vi "Dashboard Main.vi"() -> ()   [LabVIEW 2018]
uses:
  <vilib>/Utility/miscctls.llb/LVRowAndColumnTypeDef.ctl
  <vilib>/event_ctls.llb/eventvkey.ctl
  <vilib>/Rock Robotics/WPI/Dashboard/WPI_DashboardLogging Global.vi
panel:
  in  "Camera Settings Right":T1={"Frame Rate"=30, "Compression"=30, "Size"=1, "DB Camera Config"=FALSE} {"Frame Rate" scale=1.0..30.0; "Compression" scale=100.0..-1.0; "Size" items=["640x480", "320x240", "160x120"]}
  in  "Camera Name Right":string(combo)="No Camera Selection"
  out "Camera Perf":string
  in  "Camera Settings":T1={"Frame Rate"=30, "Compression"=30, "Size"=1, "DB Camera Config"=FALSE} {"Frame Rate" scale=1.0..30.0; "Compression" scale=100.0..-1.0; "Size" items=["640x480", "320x240", "160x120"]}
  in  "TCP":refnum<k5>
  in  "Rec Mode":enum32{"Stop", "Record", "Playback"}(radio)
  out "Robot IP":string
  out "Image Message":string="Timeout in Camera Communications"
  in  "Dashboard Tab":T2(tab)
  in  "Select Auto":string(combo)="Select Autonomous ..."
  out "NT Connection":bool
  out "Mode":T3(ring)=enum."Auto Disabled"
  out "Right Camera Perf":cluster{"Bandwidth (Mbps)":dbl, "FPS":dbl}
  out "Camera Image Right":T4(plugin-control)
  in  "DB/String 9":string
  in  "DB/String 8":string
  in  "DB/String 7":string
  in  "DB/String 6":string
  in  "DB/String 5":string
  in  "DB/String 4":string
  in  "DB/String 3":string
  in  "DB/String 2":string
  in  "DB/String 1":string
  in  "DB/String 0":string
  in  "DB/Slider 0":dbl(slide) scale=0.0..5.0
  in  "DB/Slider 1":dbl(slide) scale=0.0..5.0
  in  "DB/Slider 2":dbl(slide) scale=0.0..5.0
  in  "DB/Slider 3":dbl(slide) scale=0.0..5.0
  out "DB/LED 3":bool
  out "DB/LED 2":bool
  out "DB/LED 1":bool
  out "DB/LED 0":bool
  in  "DB/Button 3":bool
  in  "DB/Button 2":bool
  in  "DB/Button 1":bool
  in  "DB/Button 0":bool caption="New Name"
  in  "Test Slider":dbl(slide) scale=0.0..100.0 scale format="%#_3g"
  in  "On/Off":bool caption="Solenoid"
  in  "Test Name":u16(ring) items=["Select the test to run..."]
  in  "Test Tree":string(tree)
  in  "Motor":cluster{"Value":dbl, "Enable":bool} {"Value" scale=-1.0..1.0 scale format="%#_3g"}
  out "Progress":T5 {"Test Progress" scale=0.0..100.0}
  in  "Rev/Fwd":cluster{"Forward":bool, "Reverse":bool}
  in  "Test Ring":u16(ring) items=["Monochrome", "Color"]
  out "Cmd Status":string
  in  "Execute Command":bool
  in  "Command Params":string[][](table)
  in  "Command Selection":i32(listbox)
  in  "CheckList":i32(listbox)
  out "Tree":string(tree)
  out "Camera Image":T4(plugin-control)
  out "Background":bool
  in  "Camera Name":string(combo)="No Camera Selection"
  # "HW"
  # "HW"
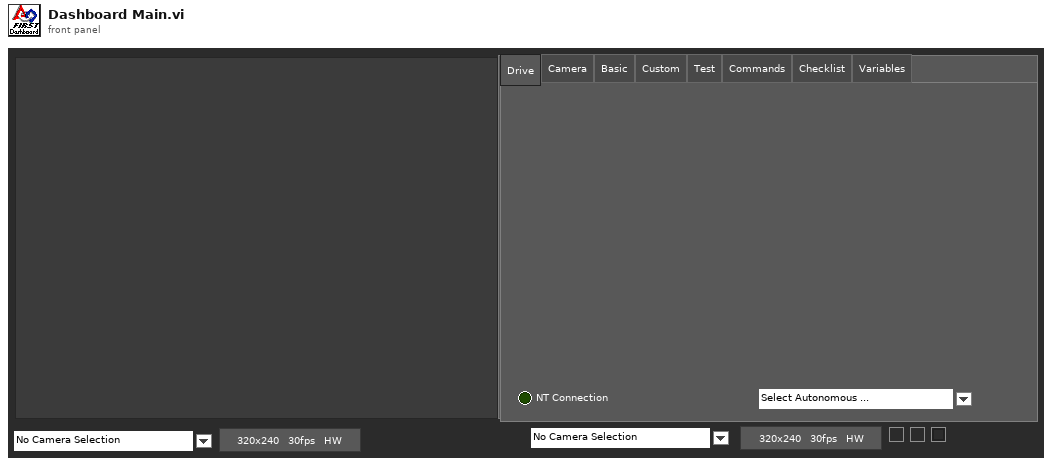
[diagram p1: front panel]
types:
  T1 = cluster{"Frame Rate":i32, "Compression":i32, "Size":u16, "DB Camera Config":bool}
  T2 = enum32{"Drive", "Camera", "Basic", "Custom", "Test", "Commands", "Checklist", "Variables"}
  T3 = enum8{"Tele-Op Disabled", "Tele-Op Enabled", "Auto Disabled", "Auto Enabled", "Test Disabled", "Test Enabled", "Disconnected", "No Code", "E-Stop"}
  T4 = typedef "IMAQ Image.ctl" = refnum<image>
  T5 = cluster{"Test Progress":u8, "Test Progress Text":string}
  T6 = cluster{"Save Path":path, "Interval (s)":dbl, "Keep":i32}
  T7 = typedef "Image Type" = u32
  T8 = cluster{"IDs":cluster{"RPC field ID":u16, "Unique ID":u16}, "String":string}
  T9 = cluster{"Error Strings":string, "Disable Counts":cluster{u16, u16}, "Rail Faults":cluster{u16, u16, u16}, "Robot IP":string, "DB Mode":u8, "Event Info":cluster{"Name":string, "Type":u8, "Number":u16, "Replay":u8}}
  T10 = cluster{"Storage":cluster{"Disk Free":u64, "RAM Block":u32, "RAM free":u32}, "CPU Utilization":cluster{"CPU % ISR":sgl, "CPU % Time Crit":sgl, "CPU % Timed Str":sgl, "CPU % High":sgl, "CPU % Above":sgl, "CPU % Normal":sgl, "CPU % Low":sgl}, "CAN":cluster{"% Bus Utilization":sgl, "Bus Off Cnt":u32, "TX_FIFO Full Cnt":u32, "Receive Error Cnt":u8, "Transmit Error Cnt":u8}, "HID":cluster{"HID Outputs":u32, "Rumble Low":u16, "Rumble High":u16}[]}
  T11 = cluster{"Status bits":cluster{"Test Mode":bool, "Autonomous":bool, "Enabled":bool, "Code Start":bool, "Brownout":bool, "Reserved 2":bool, "Reserved 3":bool, "E-Stop":bool}, "Code Trace":cluster{"Disabled":bool, "TeleOp":bool, "Auto":bool, "Test":bool}, "Controller Type":enum16{"unknown", "cRIO", "roboRio"}, "Code?":enum16{"unknown", "noCode", "code"}, "Battery V":dbl}
  T12 = cluster{"Control Bits":cluster{"TestMode":bool, "Autonomous":bool, "Enabled":bool, "FMS Present":bool, bool, bool, bool, "E-Stop":bool}, "Team Station ":u8, "Countdown":sgl, "Joystick Values":cluster{"Axes":dbl[], "Buttons":bool[], "POVs":i16[]}[]}
  T13 = cluster{"Camera Image":refnum<vi>, "Dashboard Tab":refnum<vi>, "Background":refnum<vi>, "Rec Mode":refnum<vi>, "Test Slider":refnum<vi>, "On/Off ":refnum<vi>, "Test Ring":refnum<vi>, "Rev/Fwd":refnum<vi>, "Test Name":refnum<vi>, "Motor":refnum<vi>, "Progress":refnum<vi>, "CheckList":refnum<vi>, "Tree":refnum<vi>, "Test Tree":refnum<vi>, "Command Params":refnum<vi>, "Command Selection":refnum<vi>, "Execute Command":refnum<vi>, "Cmd Status":refnum<vi>, "Camera Settings":refnum<vi>, "Camera Name":refnum<vi>, "Camera Perf":refnum<vi>, "Camera Settings Right":refnum<vi>, "Camera Name Right":refnum<vi>, "Camera Image Right":refnum<vi>}
  T14 = cluster{"Global Rectangle":i32[], "Contours":cluster{"Contour Type":u32, "ROI Type":u32, "Points":i32[]}[]}
  T15 = cluster{"Camera Name":string, string, "Saved DB Images Info":cluster{"Save Path":path, "Interval (s)":dbl, "Keep":i32}}
  T16 = cluster{"Camera Name Right":string, string, "Saved DB Images Info":cluster{"Save Path":path, "Interval (s)":dbl, "Keep":i32}}
  T17 = cluster{"Operation":enum16{"Update", "Clear"}, "Color Box":u32}[]
  T18 = typedef "eventvkey.ctl" = enum16{"ASCII", "Enter", "Return", "Shift", "Ctrl", "Alt", "Cmd", "Opt", "Caps", "NumLock", "Clear", "Break", "Up", "Down", "Left", "Right", "Insert", "Delete", "Home", "End", "PageUp", "PageDown", "Escape", "Help", "Pause", "ScrollLock", "F1", "F2", "F3", "F4", "F5", "F6", "F7", "F8", "F9", "F10", "F11", "F12", "F13", "F14", "F15", "F16", "F17", "F18", "F19", "F20", "F21", "F22", "F23", "F24", "Play", "VolumeUp", "VolumeDown", "Mute", "Two Byte Char"}
  T19 = cluster{"Image Size":bool, "Image Type":bool, "Pixel Value":bool, "ROI Information":bool, "Zoom Factor":bool}
  T20 = cluster{"Operation":enum16{"Update", "Clear"}, "Color Box":u32}
  T21 = typedef "LVRowAndColumnTypeDef.ctl" = cluster{"Row":i32, "Column":i32}
  T22 = cluster{"Shift":bool, "Ctrl":bool, "Alt":bool, "Cmd":bool, "Opt":bool}
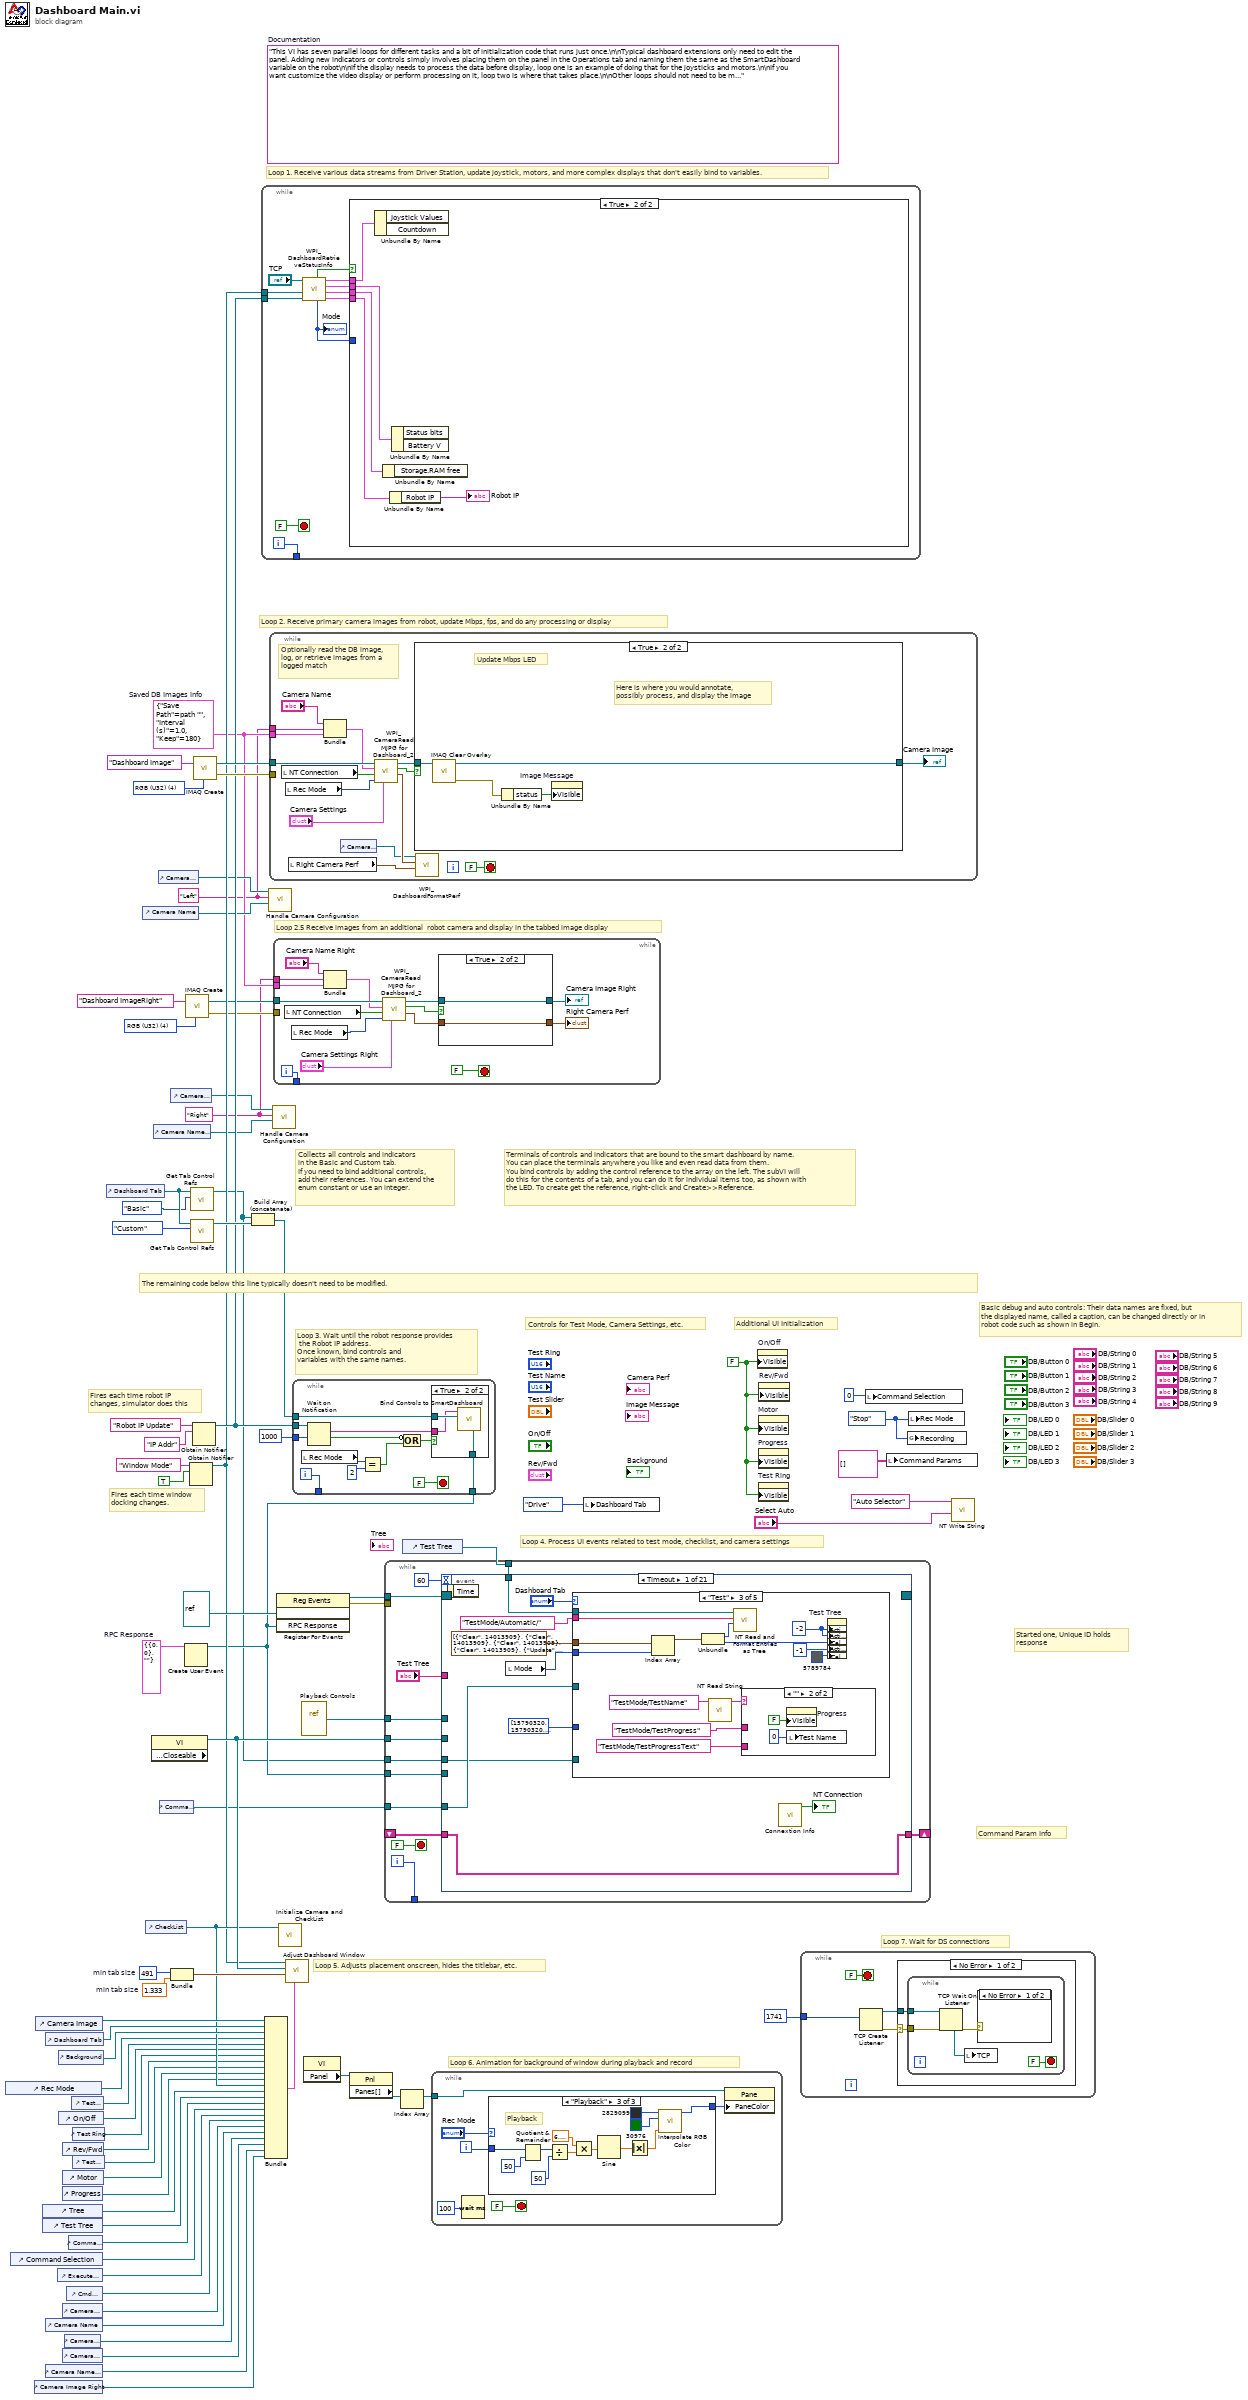
[diagram p0: block diagram]
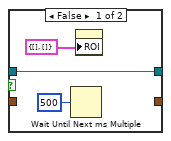
[diagram p2: hidden frame]
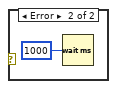
[diagram p3: hidden frame]
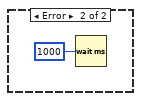
[diagram p4: hidden frame]
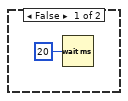
[diagram p5: hidden frame]
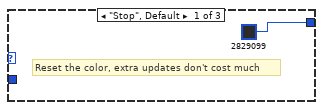
[diagram p6: hidden frame]
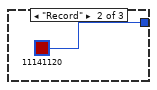
[diagram p7: hidden frame]
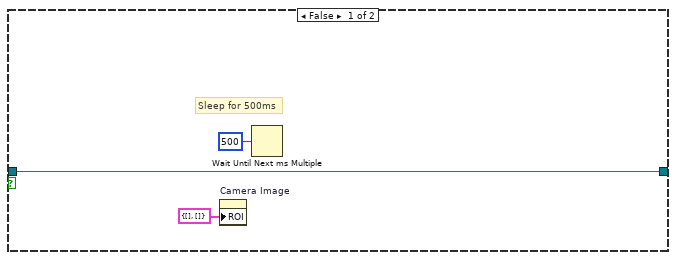
[diagram p9: hidden frame]
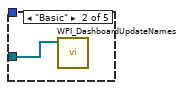
[diagram p11: hidden frame]
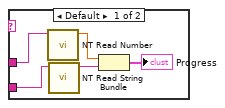
[diagram p12: hidden frame]
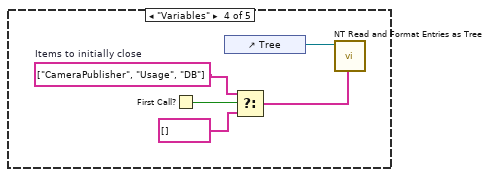
[diagram p13: hidden frame]
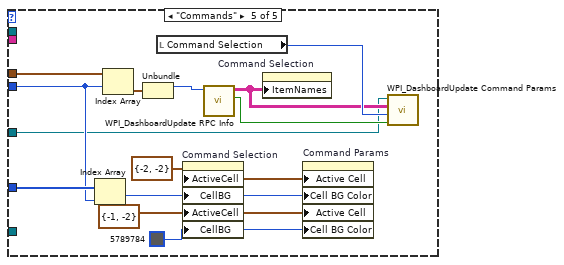
[diagram p14: hidden frame]
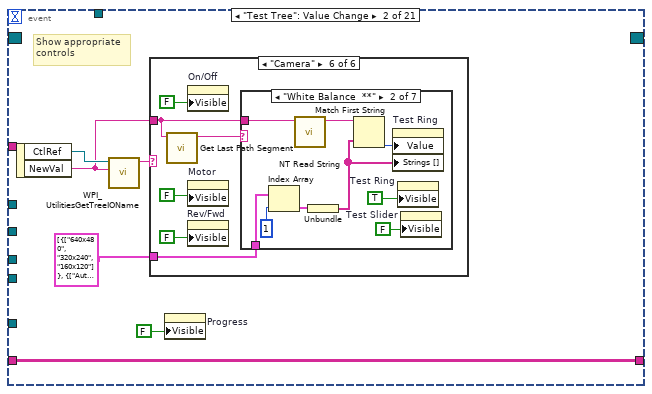
[diagram p15: hidden frame]
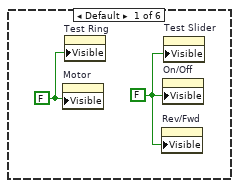
[diagram p16: hidden frame]
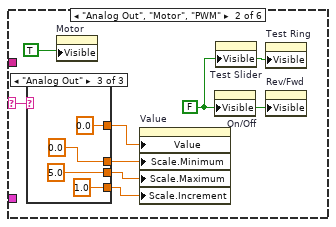
[diagram p17: hidden frame]
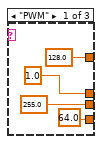
[diagram p18: hidden frame]
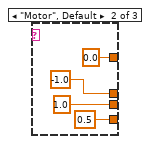
[diagram p19: hidden frame]
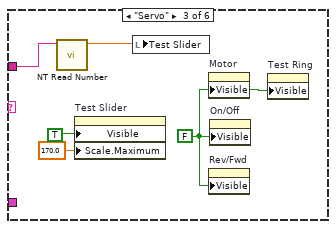
[diagram p20: hidden frame]
diagram:
  w3 = T6 {"Save Path"=path "", "Interval (s)"=1.0, "Keep"=180}  # Saved DB Images Info
  w2 = "Right"
  w1 = "Left"
  w13 = T7 4 items=["Grayscale (U8)", "Grayscale (I16)", "Grayscale (SGL)", "Complex (CSG)", "RGB (U32)", "HSL (U32)", "RGB (U64)"] ("Image Type")
  w29 = T8 {"IDs"={"RPC field ID"=0, "Unique ID"=0}, "String"=""}  # RPC Response
  w52 = 491  # min tab size
  w51 = 1.333  # min tab size
  w59 = enum32{"Stop", "Record", "Playback"}."Stop" ("Rec Mode")
  w36 = FALSE ("Visible")
  (unwired) "This VI has seven parallel loops for different tasks and a bit of initialization code that runs just once.\n\nTypical dashboard extensions only need to edit the panel. Adding new indicators or controls simply involves placing them on the panel in the Operations tab and naming them the same as the SmartDashboard variable on the robot\n\nIf the display needs to process the data before display, loop one is an example of doing that for the joysticks and motors.\n\nIf you want customize the video display or perform processing on it, loop two is where that takes place.\n\nOther loops should not need to be modified. They are pretty standard, and document the task they perform."  # Documentation
  w76 = T7 4 items=["Grayscale (U8)", "Grayscale (I16)", "Grayscale (SGL)", "Complex (CSG)", "RGB (U32)", "HSL (U32)", "RGB (U64)"] ("Image Type")
  # "Loop 2.5 Receive images from an additional  robot camera and display in the tabbed image display"
  # "Command Param Info"
  # "Started one, Unique ID holds\nresponse"
  # "Loop 7. Wait for DS connections"
  # "Basic debug and auto controls: Their data names are fixed, but\nthe displayed name, called a caption, can be changed directly or in\nrobot code such as shown in Begin."
  # "Controls for Test Mode, Camera Settings, etc."
  # "Additional UI Initialization"
  # "Loop 6. Animation for background of window during playback and record"
  # "Fires each time robot IP\nchanges, simulator does this"
  # "Fires each time window\ndocking changes."
  # "Collects all controls and indicators\nin the Basic and Custom tab.\nIf you need to bind additional controls,\nadd their references. You can extend the\nenum constant or use an integer."
  # "The remaining code below this line typically doesn't need to be modified."
  # "Loop 4. Process UI events related to test mode, checklist, and camera settings"
  # "Terminals of controls and indicators that are bound to the smart dashboard by name.\nYou can place the terminals anywhere you like and even read data from them.\nYou bind controls by adding the control reference to the array on the left. The subVI will\ndo this for the contents of a tab, and you can do it for individual items too, as shown with\nthe LED. To create get the reference, right-click and Create>>Reference."
  # "Loop 3. Wait until the robot response provides\n the Robot IP address.\nOnce known, bind controls and\nvariables with the same names."
  # "Loop 5. Adjusts placement onscreen, hides the titlebar, etc."
  # "Loop 1. Receive various data streams from Driver Station, update joystick, motors, and more complex displays that don't easily bind to variables."
  # "Loop 2. Receive primary camera images from robot, update Mbps, fps, and do any processing or display"
  n1 = control-ref of="Rec Mode"() -> (w42:refnum<vi>)
  n2 = control-ref of="Command Selection"() -> (w28:refnum<vi>)
  n3 = control-ref of="Camera Image Right"() -> (w6:refnum<vi>)
  n4 = control-ref of="Camera Image"() -> (w54:refnum<vi>)
  n5 = control-ref of="Tree"() -> (w46:refnum<vi>)
  n6 = control-ref of="Test Tree"() -> (w45:refnum<vi>)
  n7 = control-ref of="Dashboard Tab"() -> (w53:refnum<vi>)
  n8 = control-ref of="Camera Name"() -> (w19:refnum<vi>)
  n9 = control-ref of="Camera Name Right"() -> (w7:refnum<vi>)
  n10 = control-ref of="Execute Command"() -> (w30:refnum<vi>)
  n11 = control-ref of="Background"() -> (w49:refnum<vi>)
  n12 = control-ref of="On/Off"() -> (w40:refnum<vi>)
  n13 = control-ref of="Progress"() -> (w37:refnum<vi>)
  n14 = control-ref of="Camera Settings"() -> (w20:refnum<vi>)
  n15 = control-ref of="Camera Settings Right"() -> (w8:refnum<vi>)
  n16 = control-ref of="Rev/Fwd"() -> (w38:refnum<vi>)
  n17 = control-ref of="Motor"() -> (w43:refnum<vi>)
  n18 = control-ref of="Camera Perf"() -> (w18:refnum<vi>)
  n19 = control-ref of="Cmd Status"() -> (w24:refnum<vi>)
  n20 = control-ref of="Command Params"() -> (w31:refnum<vi>)
  n21 = control-ref of="Test Slider"() -> (w41:refnum<vi>)
  n22 = control-ref of="Test Ring"() -> (w39:refnum<vi>)
  n23 = control-ref of="Test Name"() -> (w44:refnum<vi>)
  n24 = control-ref of="Dashboard Tab"() -> (w57:refnum<vi>)
  n25 = control-ref of="Camera Name"() -> (w21:refnum<vi>)
  n26 = control-ref of="CheckList"() -> (w47:refnum<vi>)
  n27 = property class="VI" props=["Front Panel.Closeable"]() -> (reference out=w58:refnum<vi>)  [unwired: 2 in, 2 out]
  n28 = control-ref of="Camera Name Right"() -> (w9:refnum<vi>)
  n29 = control-ref of="Camera Settings"() -> (w22:refnum<vi>)
  n30 = control-ref of="Command Params"() -> (w23:refnum<vi>)
  n31 = control-ref of="Camera Settings Right"() -> (w10:refnum<vi>)
  n32 = Bundle("min tab size"=w52, "min tab size"=w51) -> (w50:cluster{"min tab size":i32, "min tab size":dbl})  [unwired: 1 in]
  n33 = Create User Event(user event datatype=w29) -> (user event=w25:refnum<user-event>)  [unwired: 1 in, 1 out]
  n34 = call "IMAQ Create"("Image Name"="Dashboard ImageRight", "Image Type"=w13) -> ("New Image"=w12:T4, "error out"=w11:errorcluster)  [unwired: 2 in, 1 out]
  n35 = Obtain Notifier(name (unnamed)="Window Mode", notification data type=TRUE) -> (notifier out=w34:refnum<notifier>)  [unwired: 2 in, 2 out]
  n36 = call <vilib>:"Get Tab Control Refs.vi"("Page Index"=T2."Basic" ("Dashboard Tab"), "TabControl in"=w57) -> ("ControlsOnPage"=w17:refnum<vi>[])  [unwired: 9 in]
  n37 = call <vilib>:"Get Tab Control Refs.vi"("Page Index"=T2."Custom" ("Dashboard Tab"), "TabControl in"=w57) -> ("ControlsOnPage"=w56:refnum<vi>[])  [unwired: 9 in]
  n38 = Obtain Notifier(name (unnamed)="Robot IP Update", notification data type="IP Addr" ("name (unnamed)")) -> (notifier out=w35:refnum<notifier>)  [unwired: 2 in, 2 out]
  n39 = call "IMAQ Create"("Image Name"="Dashboard Image", "Image Type"=w76) -> ("New Image"=w74:T4, "error out"=w73:errorcluster)  [unwired: 2 in, 1 out]
  n40 = Build Array (concatenate)(w17, w56) -> (w55:refnum<vi>[])
  n41 = while {
    tunnel: [w86] -> _
    tunnel: w35 -> [w80]
    tunnel: w34 -> [w77]
    i -> [w86]
    stop <- FALSE stop-if-true
    n42 = call <vilib>:"WPI_DashboardRetrieveStatusInfo.vi"("Binding Refnum"=w80, "Window Mode Notifier"=w77, "TCP Cnx"="TCP") -> ("Power and Errors"=w81:T9, "Robot Metrics"=w84:T10, "Status Info"=w85:T11, "Control Info"=w82:T12, "Robot Mode"=w79:T3, "Process?"=w83:bool)  [unwired: 3 in]
    "Mode" <- w79
    n43 = case shown="True" w83 {
      tunnel: w85 -> [_ w93]
      tunnel: w84 -> [_ w92]
      tunnel: w82 -> [_ w91]
      tunnel: w81 -> [_ w90]
      tunnel: w79 -> [_ _]
      frame False {
        n44 = Wait (ms)(milliseconds to wait=u32 20) -> ()  [unwired: 1 out]
      }
      frame True {
        n45 = Unbundle By Name(w91) -> ()  [unwired: 2 out]
        n46 = Unbundle By Name(w92) -> ()  [unwired: 1 out]
        n47 = Unbundle By Name(w90) -> ("Robot IP"=→"Robot IP":string)
        n48 = Unbundle By Name(w93) -> ()  [unwired: 2 out]
      }
    }
  }
  n49 = Bundle("Camera Image"=w54, "Dashboard Tab"=w53, "Background"=w49, "Rec Mode"=w42, "Test Slider"=w41, "On/Off"=w40, "Test Ring"=w39, "Rev/Fwd"=w38, "Test Name"=w44, "Motor"=w43, "Progress"=w37, "CheckList"=w47, "Tree"=w46, "Test Tree"=w45, "Command Params"=w31, "Command Selection"=w28, "Execute Command"=w30, "Cmd Status"=w24, "Camera Settings"=w20, "Camera Name"=w19, "Camera Perf"=w18, "Camera Settings Right"=w8, "Camera Name Right"=w7, "Camera Image Right"=w6) -> (w48:T13)  [unwired: 1 in]
  n50 = call "Handle Camera Configuration.vi"("CameraNameRef"=w21, "Display Name"=w1, "ClusterRef"=w22) -> ()  [unwired: 9 in]
  n51 = while {
    tunnel: w74 -> [w107]
    tunnel: w73 -> [_]
    tunnel: w3 -> [w100]
    tunnel: w1 -> [w97]
    stop <- FALSE stop-if-true
    # "Optionally read the DB image,\nlog, or retrieve images from a\nlogged match"
    n52 = local read "NT Connection"() -> (w101:bool)
    n53 = local read "Rec Mode"() -> (w104:enum32{"Stop", "Record", "Playback"})
    n54 = local read "Right Camera Perf"() -> (w95:cluster{"Bandwidth (Mbps)":dbl, "FPS":dbl})
    n55 = Bundle("Camera Name"="Camera Name", w97, "Saved DB Images Info"=w100) -> (w99:T15)  [unwired: 1 in]
    n56 = control-ref of="Camera Perf"() -> (w94:refnum<vi>)
    n57 = call <vilib>:"WPI_CameraRead MJPG for Dashboard_2.vi"("Camera Settings"="Camera Settings", "Rec Mode"=w104, "NT Connection"=w101, "Capture Info"=w99, "Image in"=w107) -> ("perf info"=w96:cluster{"Bandwidth (Mbps)":dbl, "fps":dbl}, "Active"=w105:bool, "Image\\ out"=w106:T4)  [unwired: 4 in]
    n58 = case shown="True" w105 {
      tunnel: w106 -> [w110 w113]
      tunnel: [w110 w112] -> w102
      frame False {
        # "Sleep for 500ms"
        n59 = property on="Camera Image" class="ImageControl"("ROI"=T14 {"Global Rectangle"=[], "Contours"=[]}) -> ()  [unwired: 2 in, 2 out]
        n60 = Wait Until Next ms Multiple(millisecond multiple=u32 500) -> ()  [unwired: 1 out]
      }
      frame True {
        # "Here is where you would annotate,\npossibly process, and display the image"
        # "Update Mbps LED"
        n61 = call "IMAQ Clear Overlay"("Image"=w113) -> ("error out"=w114:errorcluster, "Image Out"=w112:T4)  [unwired: 2 in, 7 out]
        n62 = Unbundle By Name(w114) -> ("status"=w115:bool)
        n63 = property on="Image Message" class="Str"("Visible"=w115) -> ()  [unwired: 2 in, 2 out]
      }
    }
    "Camera Image" <- w102
    n64 = call <vilib>:"WPI_DashboardFormatPerf.vi"("Right Camera Perf"=w95, "Performance"=w96, "String in"=w94) -> ()  [unwired: 9 in]
  }
  n65 = call "Handle Camera Configuration.vi"("CameraNameRef"=w9, "Display Name"=w2, "ClusterRef"=w10) -> ()  [unwired: 9 in]
  n66 = while {
    tunnel: w12 -> [w130]
    tunnel: w11 -> [_]
    tunnel: [w125] -> _
    tunnel: w3 -> [w121]
    tunnel: w2 -> [w118]
    i -> [w125]
    stop <- FALSE stop-if-true
    n67 = local read "NT Connection"() -> (w122:bool)
    n68 = local read "Rec Mode"() -> (w129:enum32{"Stop", "Record", "Playback"})
    n69 = Bundle("Camera Name Right"="Camera Name Right", w118, "Saved DB Images Info"=w121) -> (w120:T16)  [unwired: 1 in]
    n70 = call <vilib>:"WPI_CameraRead MJPG for Dashboard_2.vi"("Camera Settings"="Camera Settings Right", "Rec Mode"=w129, "NT Connection"=w122, "Capture Info"=w120, "Image in"=w130) -> ("perf info"=w116:cluster{"Bandwidth (Mbps)":dbl, "fps":dbl}, "Active"=w124:bool, "Image\\ out"=w127:T4)  [unwired: 4 in]
    n71 = case shown="True" w124 {
      tunnel: w127 -> [w132 w135]
      tunnel: [w132 w135] -> w123
      tunnel: [_ w134] -> w117
      tunnel: w116 -> [_ w134]
      frame False {
        n72 = Wait Until Next ms Multiple(millisecond multiple=u32 500) -> ()  [unwired: 1 out]
        n73 = property on="Camera Image Right" class="ImageControl"("ROI"=T14 {"Global Rectangle"=[], "Contours"=[]}) -> ()  [unwired: 2 in, 2 out]
      }
      frame True {
      }
    }
    "Camera Image Right" <- w123
    "Right Camera Perf" <- w117
  }
  n74 = register-events(refnum<vi> refnum, w25) -> (reference out=w63:refnum<event-registration>, error out=w62:errorcluster)  [unwired: 2 in]
  n75 = call "Initialize Camera and CheckList.vi"("ListBox in"=w47) -> ()  [unwired: 11 in]
  n76 = call "Adjust Dashboard Window.vi"("Sizing Refnums"=w48, "Size Constraints"=w50, "VI"=w58, "WIn Mode"=w34) -> ()  [unwired: 8 in]
  n77 = while {
    tunnel: w55 -> [w147]
    tunnel: w35 -> [w145]
    tunnel: [w143] -> _
    tunnel: u32 1000 ("milliseconds to wait") -> [w142]
    tunnel: w25 -> [w136]
    i -> [w143]
    stop <- FALSE stop-if-true
    n78 = local read "Rec Mode"() -> (w138:enum32{"Stop", "Record", "Playback"})
    n79 = Wait on Notification(notifier=w145, timeout in ms (-1)=w142) -> (notification=w144:string, timed out?=w140:bool)  [unwired: 2 in, 2 out]
    n80 = Equal?(x=w138, y=u16 2 ("Rec Mode")) -> (x = y?=w139:bool)
    n81 = Compound Arithmetic op=OR(invert w140, w139) -> (w141:bool)
    n82 = case shown="True" w141 {
      tunnel: w147 -> [_ w150]
      tunnel: w144 -> [_ w149]
      tunnel: w136 -> [_ w148]
      frame False {
      }
      frame True {
        n83 = call <vilib>:"Bind Controls to SmartDashboard.vi"("RPC ref"=w148, "Bound Control Refs"=w150, "Server IP Address"=w149) -> ()  [unwired: 9 in]
      }
    }
  }
  n84 = vi-ref "Playback Controls.vi"() -> (w64:refnum<vi>)
  n85 = property class="VI"() -> ("Panel"=w66:refnum<vi>)  [unwired: 2 in, 2 out]
  n86 = property class="Pnl"(reference=w66) -> ("Panes[]"=w67:refnum<vi>[])  [unwired: 1 in, 2 out]
  n87 = Index Array(array=w67) -> (element=w65:refnum<vi>)  [unwired: 1 in]
  n88 = control-ref of="Test Tree"() -> (w68:refnum<vi>)
  n89 = while {
    tunnel: [w160] -> _
    tunnel: w68 -> [w159]
    tunnel: w64 -> [w158]
    tunnel: w63 -> [w157]
    tunnel: w62 -> [_]
    tunnel: w58 -> [w156]
    tunnel: w25 -> [w155]
    tunnel: w23 -> [w154]
    shift-right: [w153] -> _
    shift-left: _ -> [w152]
    tunnel: w17 -> [w151]
    i -> [w160]
    stop <- FALSE stop-if-true
    n90 = event shown="[0] Timeout" {
      selector: w157 -> [_ _ _ _ _ _ _ _ _ _ _ _ _ _ _ _ _ _ _ _ _]
      dyn-events: [_ _ _ _ _ _ _ _ _ _ _ _ _ _ _ _ w420 _ _ _ _] -> _
      timeout: u32 60 ("milliseconds to wait") -> [_ _ _ _ _ _ _ _ _ _ _ _ _ _ _ _ _ _ _ _ _]
      tunnel: w159 -> [w172 _ _ _ _ _ _ _ _ _ _ _ _ _ _ _ _ _ _ _ _]
      tunnel: "Test Tree" -> [_ _ _ _ _ _ _ _ _ _ _ w387 w395 w397 w401 w409 _ _ _ _ _]
      tunnel: w158 -> [_ _ _ _ _ _ _ _ _ _ _ _ _ _ _ _ w422 _ w440 _ _]
      tunnel: w156 -> [_ _ _ _ _ _ _ _ _ _ _ _ _ _ _ _ w418 _ _ _ _]
      tunnel: w155 -> [_ _ _ _ _ _ _ _ _ _ _ _ _ _ _ _ w416 _ _ _ _]
      tunnel: w154 -> [w167 _ _ _ _ _ w338 _ _ _ _ _ _ _ _ _ _ _ _ _ _]
      tunnel: [w166 w215 w317 w322 w331 w335 w336 w345 w355 w362 w374 w386 w393 w396 w400 w408 w415 w435 w437 w441 w454] -> w153
      tunnel: w152 -> [w166 w215 w317 w322 w331 w335 w336 _ _ w362 w374 w386 w393 w396 w400 w408 w415 w435 w437 w441 w454]
      tunnel: w151 -> [w164 _ _ _ _ _ _ _ _ _ _ _ _ _ _ _ _ _ _ _ _]
      event Timeout {
        n91 = event-data() -> ()  [unwired: 1 in, 1 out]
        n92 = local read "Mode"() -> (w169:T3)
        n93 = case shown="\"Test\"" "Dashboard Tab" {
          tunnel: w172 -> [_ _ w188 _ _]
          tunnel: "TestMode/Automatic/" ("Name Pattern") -> [_ _ w187 _ _]
          tunnel: T17 [{"Operation"=enum."Clear", "Color Box"=14013909}, {"Operation"=enum."Clear", "Color Box"=14013909}, {"Operation"=enum."Clear", "Color Box"=14013909}, {"Operation"=enum."Clear", "Color Box"=14013909}, {"Operation"=enum."Update", "Color Box"=14013909}, {"Operation"=enum."Update", "Color Box"=16777215}, {"Operation"=enum."Clear", "Color Box"=14013909}, {"Operation"=enum."Clear", "Color Box"=14013909}, {"Operation"=enum."Clear", "Color Box"=14013909}] -> [_ _ w180 _ w208]
          tunnel: w169 -> [_ _ w179 _ w207]
          tunnel: u32[] [15790320, 15790320, 15790320, 15790320, 16777215, 16777215, 15790320, 15790320, 15790320] -> [_ _ _ _ w213]
          tunnel: w167 -> [_ _ _ _ w201]
          tunnel: w164 -> [_ w174 _ _ _]
          frame "Custom", Default {
          }
          frame "Basic" {
            n94 = call <vilib>:"WPI_DashboardUpdateNames.vi"("Controls on Tab"=w174) -> ()  [unwired: 11 in]
          }
          frame "Test" {
            w186 = -2 ("Active Item:Row Number")
            n95 = Index Array(array=w180, index=w179) -> (element=w181:T20)
            n96 = Unbundle(w181) -> ("Operation"=w182:enum16{"Update", "Clear"}, "Color Box"=w183:u32)
            n97 = call <vilib>:"NT Read String.vi"("Name"="TestMode/TestName") -> ("String"=w177:string)  [unwired: 9 in, 1 out]
            n98 = call <vilib>:"NT Read and Format Entries as Tree.vi"("Operation"=w182, "Name Pattern"=w187, "Tree Refnum"=w188) -> ()  [unwired: 7 in, 2 out]
            n99 = case shown="\"\"" w177 {
              tunnel: "TestMode/TestProgress" ("Name") -> [w190 _]
              tunnel: "TestMode/TestProgressText" ("Name") -> [w189 _]
              frame Default {
                n100 = call <vilib>:"NT Read Number.vi"("Name"=w190) -> ("Numeric"=w191:dbl)  [unwired: 9 in, 1 out]
                n101 = call <vilib>:"NT Read String.vi"("Name"=w189) -> ("String"=w192:string)  [unwired: 9 in, 1 out]
                n102 = Bundle("Numeric"=w191, "String"=w192) -> (→"Progress":cluster{"Numeric":dbl, "String":string})  [unwired: 1 in]
              }
              frame "" {
                n103 = property on="Progress" class="Clust (strict)"("Visible"=FALSE) -> ()  [unwired: 2 in, 2 out]
                n104 = local write "Test Name"(u16 0) -> ()
              }
            }
            n105 = property on="Test Tree" class="Tree (strict)"("Active Item Row Number"=w186, "ActiveColNum"=w186, "CellBG"=w183, "Active Item Row Number"=-1 ("Active Item:Row Number"), "CellBG"=u32 5789784 ("Color Box")) -> ()  [unwired: 2 in, 2 out]
          }
          frame "Variables" {
            w198 = string[] ["CameraPublisher", "Usage", "DB"]  # Items to initially close
            n106 = First Call?() -> (First Call?: T/F=w199:bool)
            n107 = control-ref of="Tree"() -> (w200:refnum<vi>)
            n108 = Select(t=w198, s=w199, f=string[] []) -> (s? t:f=w196:string[])
            n109 = call <vilib>:"NT Read and Format Entries as Tree.vi"("Tags to  Close"=w196, "Tree Refnum"=w200) -> ()  [unwired: 8 in, 2 out]
          }
          frame "Commands" {
            w209 = u32 5789784 ("Color Box")
            w210 = T21 {"Row"=-1, "Column"=-2} ("Active Cell:Active Cell")
            w212 = T21 {"Row"=-2, "Column"=-2} ("Active Cell:Active Cell")
            n110 = Index Array(array=w213, index=w207) -> (element=w211:u32)
            n111 = Index Array(array=w208, index=w207) -> (element=w206:T20)
            n112 = Unbundle(w206) -> ("Operation"=w205:enum16{"Update", "Clear"})  [unwired: 1 out]
            n113 = local read "Command Selection"() -> (w204:i32)
            n114 = property on="Command Selection" class="MCListbox (strict)"("ActiveCell"=w212, "CellBG"=w211, "ActiveCell"=w210, "CellBG"=w209) -> ()  [unwired: 2 in, 2 out]
            n115 = call <vilib>:"WPI_DashboardUpdate RPC Info.vi"("Operation"=w205) -> ("update"=w203:bool, "commands"=w202:string[][])  [unwired: 9 in]
            n116 = property on="Command Selection" class="MCListbox (strict)"("ItemNames"=w202) -> ()  [unwired: 2 in, 2 out]
            n117 = property on="Command Params" class="Tbl (strict)"("Active Cell"=w212, "Cell BG Color"=w211, "Active Cell"=w210, "Cell BG Color"=w209) -> ()  [unwired: 2 in, 2 out]
            n118 = call <vilib>:"WPI_DashboardUpdate Command Params.vi"("Update"=w203, "NewVal"=w204, "Commands"=w202, "Param Tbl"=w201) -> ()  [unwired: 7 in, 1 out]
          }
        }
        n119 = call <vilib>:"Connextion Info.vi"() -> ("Connected"=→"NT Connection":bool)  [unwired: 10 in, 1 out]
      }
      event "Test Tree": Value Change {
        # "Show appropriate\ncontrols"
        n120 = event-data() -> ("CtlRef"=w218:refnum<vi>, "NewVal"=w216:string)  [unwired: 1 in]
        n121 = call <vilib>:"WPI_UtilitiesGetTreeIOName.vi"("NewVal"=w216, "TreeControl in"=w218) -> ("I/O Name"=w219:string)  [unwired: 9 in]
        n122 = case shown="\"Camera\"" w219 {
          selector: w219 -> [_ w226 _ w248 w257 _]
          tunnel: w216 -> [_ _ w245 w247 _ w264]
          tunnel: cluster{string[]}[] [{["640x480", "320x240", "160x120"]}, {["Auto", "Fixed indoor", "Fixed outdoor 1", "Fixed outdoor 2", "Fixed fluorescent 1", "Fixed fluorescent 2", "Hold current"]}, {["Auto", "Flicker-free 50 Hz", "Flicker-free 60 Hz", "Hold current"]}, {["None", "Prioritize frame rate", "Prioritize image quality"]}, {["Monochrome", "Color"]}] -> [_ _ _ _ _ w263]
          frame Default {
            w221 = FALSE ("Visible")
            w220 = FALSE ("Visible")
            n123 = property on="Motor" class="Clust (strict)"("Visible"=w220) -> ()  [unwired: 2 in, 2 out]
            n124 = property on="Test Ring" class="Ring (strict)"("Visible"=w220) -> ()  [unwired: 2 in, 2 out]
            n125 = property on="Rev/Fwd" class="Clust (strict)"("Visible"=w221) -> ()  [unwired: 2 in, 2 out]
            n126 = property on="On/Off" class="Bool (strict)"("Visible"=w221) -> ()  [unwired: 2 in, 2 out]
            n127 = property on="Test Slider" class="Slide (strict)"("Visible"=w221) -> ()  [unwired: 2 in, 2 out]
          }
          frame "Analog Out", "Motor", "PWM" {
            w227 = FALSE ("Visible")
            n128 = case shown="\"Analog Out\"" w226 {
              tunnel: [1.0 ("Value") -1.0 ("Value") 0.0 ("Value")] -> w225
              tunnel: [255.0 ("Value") 1.0 ("Value") 5.0 ("Value")] -> w224
              tunnel: [128.0 ("Value") 0.0 ("Value") 0.0 ("Value")] -> w223
              tunnel: [64.0 ("Value") 0.5 ("Value") 1.0 ("Value")] -> w222
              frame "PWM" {
              }
              frame "Motor", Default {
              }
              frame "Analog Out" {
              }
            }
            n129 = property on="Motor" class="Clust (strict)"("Visible"=TRUE) -> ()  [unwired: 2 in, 2 out]
            n130 = property on="Value" class="Slide (strict)"("Value"=w223, "Scale.Minimum"=w225, "Scale.Maximum"=w224, "Scale.Increment"=w222) -> ()  [unwired: 2 in, 2 out]
            n131 = property on="On/Off" class="Bool (strict)"("Visible"=w227) -> ()  [unwired: 2 in, 2 out]
            n132 = property on="Test Slider" class="Slide (strict)"("Visible"=w227) -> ()  [unwired: 2 in, 2 out]
            n133 = property on="Test Ring" class="Ring (strict)"("Visible"=w227) -> ()  [unwired: 2 in, 2 out]
            n134 = property on="Rev/Fwd" class="Clust (strict)"("Visible"=w227) -> ()  [unwired: 2 in, 2 out]
          }
          frame "Servo" {
            w243 = FALSE ("Visible")
            n135 = call <vilib>:"NT Read Number.vi"("Name"=w245) -> ("Numeric"=w244:dbl)  [unwired: 9 in, 1 out]
            n136 = property on="Test Slider" class="Slide (strict)"("Visible"=TRUE, "Scale.Maximum"=170.0 ("Scale.Range:Maximum")) -> ()  [unwired: 2 in, 2 out]
            n137 = local write "Test Slider"(w244) -> ()
            n138 = property on="Motor" class="Clust (strict)"("Visible"=w243) -> ()  [unwired: 2 in, 2 out]
            n139 = property on="Rev/Fwd" class="Clust (strict)"("Visible"=w243) -> ()  [unwired: 2 in, 2 out]
            n140 = property on="On/Off" class="Bool (strict)"("Visible"=w243) -> ()  [unwired: 2 in, 2 out]
            n141 = property on="Test Ring" class="Ring (strict)"("Visible"=w243) -> ()  [unwired: 2 in, 2 out]
          }
          frame "Relay", "Solenoid" {
            w246 = FALSE ("Visible")
            n142 = property on="Motor" class="Clust (strict)"("Visible"=w246) -> ()  [unwired: 2 in, 2 out]
            n143 = property on="Test Slider" class="Slide (strict)"("Visible"=w246) -> ()  [unwired: 2 in, 2 out]
            n144 = Search and Replace String(input string=w247, search string="/Value  **", replace string="/Direction") -> (result string=w253:string)  [unwired: 5 in, 3 out]
            n145 = property on="Test Ring" class="Ring (strict)"("Visible"=w246) -> ()  [unwired: 2 in, 2 out]
            n146 = call <vilib>:"NT Read String.vi"("Name"=w253) -> ("String"=w251:string)  [unwired: 9 in, 1 out]
            n147 = Equal?(x="Both directions", y=w251) -> (x = y?=w249:bool)
            n148 = Not(x=w249) -> (.not. x?=w250:bool)
            n149 = property on="Rev/Fwd" class="Clust (strict)"("Visible"=w249) -> ()  [unwired: 2 in, 2 out]
            n150 = property on="On/Off" class="Bool (strict)"("Visible"=w250, "Caption.Text"=w248) -> ()  [unwired: 2 in, 2 out]
          }
          frame "Compressor", "Digital Out" {
            w256 = FALSE ("Visible")
            # "Get direction and finish"
            n151 = property on="Motor" class="Clust (strict)"("Visible"=w256) -> ()  [unwired: 2 in, 2 out]
            n152 = property on="Test Slider" class="Slide (strict)"("Visible"=w256) -> ()  [unwired: 2 in, 2 out]
            n153 = property on="Test Ring" class="Ring (strict)"("Visible"=w256) -> ()  [unwired: 2 in, 2 out]
            n154 = property on="On/Off" class="Bool (strict)"("Visible"=TRUE, "Caption.Text"=w257) -> ()  [unwired: 2 in, 2 out]
            n155 = property on="Rev/Fwd" class="Clust (strict)"("Visible"=FALSE) -> ()  [unwired: 2 in, 2 out]
          }
          frame "Camera" {
            n156 = call <vilib>:"Get Last Path Segment.vi"("String in"=w264) -> ("String out"=w265:string)  [unwired: 10 in]
            n157 = property on="On/Off" class="Bool (strict)"("Visible"=FALSE) -> ()  [unwired: 2 in, 2 out]
            n158 = property on="Motor" class="Clust (strict)"("Visible"=FALSE) -> ()  [unwired: 2 in, 2 out]
            n159 = property on="Rev/Fwd" class="Clust (strict)"("Visible"=FALSE) -> ()  [unwired: 2 in, 2 out]
            n160 = case shown="\"White Balance  **\"" w265 {
              tunnel: w264 -> [w271 w280 w289 w298 w307 _ w313]
              tunnel: w263 -> [w269 w277 w286 w295 w304 _ _]
              frame "Size  **" {
                n161 = Index Array(array=w269) -> (element=w268:cluster{string[]})  [unwired: 1 in]
                n162 = call <vilib>:"NT Read String.vi"("Name"=w271) -> ("String"=w270:string)  [unwired: 9 in, 1 out]
                n163 = Unbundle(w268) -> (w266:string[])
                n164 = Match First String(2:w266, 3:w270) -> (0:w267:i32)  [unwired: 1 out]
                n165 = property on="Test Ring" class="Ring (strict)"("Value"=w267, "Strings []"=w266) -> ()  [unwired: 2 in, 2 out]
                n166 = property on="Test Ring" class="Ring (strict)"("Visible"=TRUE) -> ()  [unwired: 2 in, 2 out]
                n167 = property on="Test Slider" class="Slide (strict)"("Visible"=FALSE) -> ()  [unwired: 2 in, 2 out]
              }
              frame "White Balance  **" {
                n168 = Index Array(array=w277, index=1) -> (element=w278:cluster{string[]})
                n169 = call <vilib>:"NT Read String.vi"("Name"=w280) -> ("String"=w279:string)  [unwired: 9 in, 1 out]
                n170 = Unbundle(w278) -> (w275:string[])
                n171 = Match First String(2:w275, 3:w279) -> (0:w274:i32)  [unwired: 1 out]
                n172 = property on="Test Ring" class="Ring (strict)"("Value"=w274, "Strings []"=w275) -> ()  [unwired: 2 in, 2 out]
                n173 = property on="Test Ring" class="Ring (strict)"("Visible"=TRUE) -> ()  [unwired: 2 in, 2 out]
                n174 = property on="Test Slider" class="Slide (strict)"("Visible"=FALSE) -> ()  [unwired: 2 in, 2 out]
              }
              frame "Exposure  **" {
                n175 = Index Array(array=w286, index=2) -> (element=w287:cluster{string[]})
                n176 = call <vilib>:"NT Read String.vi"("Name"=w289) -> ("String"=w288:string)  [unwired: 9 in, 1 out]
                n177 = Unbundle(w287) -> (w283:string[])
                n178 = Match First String(2:w283, 3:w288) -> (0:w284:i32)  [unwired: 1 out]
                n179 = property on="Test Ring" class="Ring (strict)"("Value"=w284, "Strings []"=w283) -> ()  [unwired: 2 in, 2 out]
                n180 = property on="Test Ring" class="Ring (strict)"("Visible"=TRUE) -> ()  [unwired: 2 in, 2 out]
                n181 = property on="Test Slider" class="Slide (strict)"("Visible"=FALSE) -> ()  [unwired: 2 in, 2 out]
              }
              frame "Exposure Priority  **" {
                n182 = Index Array(array=w295, index=3) -> (element=w296:cluster{string[]})
                n183 = call <vilib>:"NT Read String.vi"("Name"=w298) -> ("String"=w297:string)  [unwired: 9 in, 1 out]
                n184 = Unbundle(w296) -> (w292:string[])
                n185 = Match First String(2:w292, 3:w297) -> (0:w293:i32)  [unwired: 1 out]
                n186 = property on="Test Ring" class="Ring (strict)"("Value"=w293, "Strings []"=w292) -> ()  [unwired: 2 in, 2 out]
                n187 = property on="Test Ring" class="Ring (strict)"("Visible"=TRUE) -> ()  [unwired: 2 in, 2 out]
                n188 = property on="Test Slider" class="Slide (strict)"("Visible"=FALSE) -> ()  [unwired: 2 in, 2 out]
              }
              frame "Color Enable  **" {
                n189 = Index Array(array=w304, index=4) -> (element=w305:cluster{string[]})
                n190 = call <vilib>:"NT Read String.vi"("Name"=w307) -> ("String"=w306:string)  [unwired: 9 in, 1 out]
                n191 = Unbundle(w305) -> (w301:string[])
                n192 = Match First String(2:w301, 3:w306) -> (0:w302:i32)  [unwired: 1 out]
                n193 = property on="Test Ring" class="Ring (strict)"("Value"=w302, "Strings []"=w301) -> ()  [unwired: 2 in, 2 out]
                n194 = property on="Test Ring" class="Ring (strict)"("Visible"=TRUE) -> ()  [unwired: 2 in, 2 out]
                n195 = property on="Test Slider" class="Slide (strict)"("Visible"=FALSE) -> ()  [unwired: 2 in, 2 out]
              }
              frame Default {
                n196 = property on="Test Ring" class="Ring (strict)"("Visible"=FALSE) -> ()  [unwired: 2 in, 2 out]
                n197 = property on="Test Slider" class="Slide (strict)"("Visible"=FALSE) -> ()  [unwired: 2 in, 2 out]
              }
              frame "Brightness  **", "Color Level  **", "Compression  **", "FPS  **", "Sharpness  **" {
                n198 = call <vilib>:"NT Read Number.vi"("Name"=w313) -> ("Numeric"=w312:dbl)  [unwired: 9 in, 1 out]
                n199 = local write "Test Slider"(w312) -> ()
                n200 = property on="Test Slider" class="Slide (strict)"("Visible"=TRUE, "Scale.Maximum"=100.0 ("Scale.Range:Maximum")) -> ()  [unwired: 2 in, 2 out]
                n201 = property on="Test Ring" class="Ring (strict)"("Visible"=FALSE) -> ()  [unwired: 2 in, 2 out]
              }
            }
          }
        }
        n202 = property on="Progress" class="Clust (strict)"("Visible"=FALSE) -> ()  [unwired: 2 in, 2 out]
      }
      event "Test Name": Mouse Enter {
        # "Populate the ring with the list of tests"
        n203 = event-data() -> ()  [unwired: 1 in, 1 out]
        n204 = call <vilib>:"NT Read String Array.vi"("Name"="TestMode/TestList") -> ("String Array"=w321:string[])  [unwired: 9 in, 1 out]
        n205 = Build Array (concatenate)("Select the test to run...", w321) -> (w320:string[])
        n206 = property on="Test Name" class="Ring (strict)"("Strings []"=w320) -> ()  [unwired: 2 in, 2 out]
      }
      event "Test Name": Value Change {
        w323 = FALSE ("Visible")
        # "Tell the robot the test name to run"
        n207 = event-data() -> ("NewVal"=w327:u16)  [unwired: 1 in]
        n208 = property on="Test Name" class="Ring (strict)"() -> ("Strings []"=w328:string[])  [unwired: 2 in, 2 out]
        n209 = local write "Progress"(T5 {"Test Progress"=0, "Test Progress Text"=""} ("Progress")) -> ()
        n210 = Index Array(array=w328, index=w327) -> (element=w326:string)
        n211 = call <vilib>:"NT Write String.vi"("String"=w326, "Name"="TestMode/TestName") -> ()  [unwired: 9 in, 1 out]
        n212 = property on="Progress" class="Clust (strict)"("Visible"=TRUE) -> ()  [unwired: 2 in, 2 out]
        n213 = property on="Motor" class="Clust (strict)"("Visible"=w323) -> ()  [unwired: 2 in, 2 out]
        n214 = property on="Test Slider" class="Slide (strict)"("Visible"=w323) -> ()  [unwired: 2 in, 2 out]
        n215 = property on="On/Off" class="Bool (strict)"("Visible"=w323) -> ()  [unwired: 2 in, 2 out]
        n216 = property on="Rev/Fwd" class="Clust (strict)"("Visible"=w323) -> ()  [unwired: 2 in, 2 out]
        n217 = property on="Test Ring" class="Ring (strict)"("Visible"=w323) -> ()  [unwired: 2 in, 2 out]
      }
      event "Select Auto": Mouse Enter {
        # "Populate the combo box with the list of autonomous options"
        n218 = event-data() -> ()  [unwired: 1 in, 1 out]
        n219 = call <vilib>:"NT Read String Array.vi"("Name"="Auto List") -> ("String Array"=w330:string[])  [unwired: 9 in, 1 out]
        n220 = property on="Select Auto" class="CmbBox"("Strings[]"=w330) -> ()  [unwired: 2 in, 2 out]
      }
      event "Select Auto": Value Change {
        # "User modified the Auto Selection. Write to NT variable so robot knows."
        n221 = event-data() -> ("NewVal"=w333:string)  [unwired: 1 in]
        n222 = call <vilib>:"NT Write String.vi"("String"=w333, "Name"="Auto Selector") -> ()  [unwired: 9 in, 1 out]
      }
      event "Command Selection": Value Change {
        # "Get the params and show in table"
        n223 = event-data() -> ("NewVal"=w339:i32)  [unwired: 1 in]
        n224 = property on="Command Selection" class="MCListbox (strict)"() -> ("ItemNames"=w337:string[][])  [unwired: 2 in, 2 out]
        n225 = call <vilib>:"WPI_DashboardUpdate Command Params.vi"("NewVal"=w339, "Commands"=w337, "Param Tbl"=w338) -> ()  [unwired: 8 in, 1 out]
      }
      event "Execute Command": Value Change {
        # "Started one, Unique ID holds\nresponse"
        n226 = event-data() -> ()  [unwired: 1 in, 1 out]
        n227 = property on="Command Selection" class="MCListbox (strict)"() -> ("ItemNames"=w350:string[][])  [unwired: 2 in, 2 out]
        n228 = Index Array(array=w350, index (row)="Command Selection", index (col)=0) -> (element=w348:string)
        n229 = call <vilib>:"Invoke Commands.vi"("Command Params"="Command Params", "Function Name"=w348) -> ("Params"=w344:u8, "Started"=w343:bool)  [unwired: 7 in, 1 out]
        n230 = Array Subset(array="Command Params", length (row)=w344) -> (w345:string[][])  [unwired: 3 in]
        n231 = Select(t="Executing" ("Cmd Status"), s=w343, f="" ("Cmd Status")) -> (s? t:f=→"Cmd Status":string)
      }
      event "Command Selection": Double Click {
        n232 = event-data() -> ("Row"=w358:i32)  [unwired: 1 in]
        n233 = property on="Command Selection" class="MCListbox (strict)"() -> ("ItemNames"=w361:string[][])  [unwired: 2 in, 2 out]
        n234 = local read "Command Params"() -> (w357:string[][])
        n235 = Index Array(array=w361, index (row)=w358, index (col)=0) -> (element=w359:string)
        n236 = call <vilib>:"Invoke Commands.vi"("Command Params"=w357, "Function Name"=w359) -> ("Params"=w356:u8, "Started"=w351:bool)  [unwired: 7 in, 1 out]
        n237 = Array Subset(array=w357, length (row)=w356) -> (w355:string[][])  [unwired: 3 in]
        n238 = Select(t="Executing" ("Cmd Status"), s=w351, f="" ("Cmd Status")) -> (s? t:f=w352:string)
        n239 = local write "Cmd Status"(w352) -> ()
      }
      event "CheckList": Double Click {
        # "Shift clears all"
        # "Update symbols on the listbox"
        n240 = event-data() -> ("PlatMods.Shift"=w363:bool, "Row"=w365:i32)  [unwired: 1 in]
        n241 = case shown="True" w363 {
          tunnel: w365 -> [w369 _]
          tunnel: 1 -> [w368 _]
          frame False {
            n242 = property on="CheckList" class="LstBox (strict)"() -> ("Item Symbols"=w367:i32[])  [unwired: 2 in, 2 out]
            n243 = Replace Array Subset(array=w367, new element=w368, index=w369) -> (w366:i32[])
            n244 = property on="CheckList" class="LstBox (strict)"("Item Symbols"=w366) -> ()  [unwired: 2 in, 2 out]
          }
          frame True {
            w370 = 0 ("Top Row")
            n245 = property on="CheckList" class="LstBox (strict)"() -> ("Number of Rows"=w372:u32)  [unwired: 2 in, 2 out]
            n246 = Initialize Array(0, w372) -> (w371:i32[])
            n247 = property on="CheckList" class="LstBox (strict)"("Top Row"=w370, "Value"=w370, "Item Symbols"=w371) -> ()  [unwired: 2 in, 2 out]
          }
        }
      }
      event "CheckList": Key Down {
        # "Update symbols on the listbox\nLeft and right keys check and uncheck"
        n248 = event-data() -> ("VKey"=w376:T18)  [unwired: 1 in]
        n249 = case shown="\"Left\", \"Right\"" w376 {
          selector: w376 -> [w381 _]
          tunnel: eventvkey."Left" ("VKey") -> [w379 _]
          frame "Left", "Right" {
            n250 = Equal?(x=w379, y=w381) -> (x = y?=w380:bool)
            n251 = Select(t=0, s=w380, f=1) -> (s? t:f=w382:i32)
            n252 = property on="CheckList" class="LstBox (strict)"() -> ("Item Symbols"=w385:i32[])  [unwired: 2 in, 2 out]
            n253 = Replace Array Subset(array=w385, new element=w382, index="CheckList") -> (w384:i32[])
            n254 = property on="CheckList" class="LstBox (strict)"("Item Symbols"=w384) -> ()  [unwired: 2 in, 2 out]
          }
          frame Default {
          }
        }
      }
      event "Motor.Enable": Value Change {
        # "When the test mode otor enable helper is set, update that\ntree row item's value"
        n255 = event-data() -> ("NewVal"=w391:bool)  [unwired: 1 in]
        n256 = Unbundle("Motor") -> ("Value"=w390:dbl)  [unwired: 1 out]
        n257 = Select(t=w390, s=w391, f=0.0) -> (s? t:f=w388:dbl)
        n258 = call <vilib>:"NT Write Number.vi"("Numeric"=w388, "Name"=w387) -> ()  [unwired: 9 in, 1 out]
      }
      event "Test Slider": Value Change {
        # "When the test mode slider helper is set, update that\ntree row item's value"
        n259 = event-data() -> ("NewVal"=w394:dbl)  [unwired: 1 in]
        n260 = call <vilib>:"NT Write Number.vi"("Numeric"=w394, "Name"=w395) -> ()  [unwired: 9 in, 1 out]
      }
      event "On/Off": Value Change {
        # "When the test mode on/off helper value is set, update that\ntree row item's value"
        n261 = event-data() -> ("NewVal"=w399:bool)  [unwired: 1 in]
        n262 = Boolean To (0,1)(Boolean=w399) -> (0, 1=w398:i16)
        n263 = call <vilib>:"NT Write Number.vi"("Numeric"=w398, "Name"=w397) -> ()  [unwired: 9 in, 1 out]
      }
      event "Rev/Fwd": Value Change {
        # "When the test mode helper value for relays is set, update that\ntree row item's value"
        n264 = event-data() -> ("NewVal.Forward"=w407:bool, "NewVal.Reverse"=w406:bool)  [unwired: 1 in]
        n265 = Boolean To (0,1)(Boolean=w407) -> (0, 1=w403:i16)
        n266 = Boolean To (0,1)(Boolean=w406) -> (0, 1=w405:i16)
        n267 = Negate(x=w405) -> (-x=w404:i16)
        n268 = Add(x=w403, y=w404) -> (x+y=w402:i16)
        n269 = call <vilib>:"NT Write Number.vi"("Numeric"=w402, "Name"=w401) -> ()  [unwired: 9 in, 1 out]
      }
      event "Test Ring": Value Change {
        # "When a test mode helper value is selected from the ring,\nset the tree item's variable to the string value"
        n270 = event-data() -> ("NewVal"=w411:u16)  [unwired: 1 in]
        n271 = property on="Test Ring" class="Ring (strict)"() -> ("Strings []"=w412:string[])  [unwired: 2 in, 2 out]
        n272 = Index Array(array=w412, index=w411) -> (element=w410:string)
        n273 = call <vilib>:"NT Write String.vi"("String"=w410, "Name"=w409) -> ()  [unwired: 9 in, 1 out]
      }
      event "Rec Mode": Value Change {
        # "Update globals for recording mode and path to read log from.\nClear when logging and let NetworkTables set path for vision to\nuse."
        n274 = event-data() -> ("NewVal"=w423:enum32{"Stop", "Record", "Playback"})  [unwired: 1 in]
        n275 = global write "WPI_DashboardLogging Global.vi" "Logging Filename"(path "") -> ()
        n276 = global write "WPI_DashboardLogging Global.vi" "Recording"(w423) -> ()
        n277 = case shown="\"Playback\"" w423 {
          tunnel: w422 -> [_ w425 w434]
          tunnel: [_ _ w433] -> w420
          tunnel: [_ _ w432] -> _
          tunnel: w418 -> [_ _ w430]
          tunnel: cluster{i32, i32} {-250, 170} -> [_ _ w429]
          tunnel: [_ _ T19 {"Image Size"=TRUE, "Image Type"=TRUE, "Pixel Value"=TRUE, "ROI Information"=TRUE, "Zoom Factor"=FALSE} ("Image Information Shown:All Elements")] -> w413
          tunnel: [_ _ TRUE ("Zoom Factor")] -> w414
          tunnel: w416 -> [_ _ w426]
          frame Default {
          }
          frame "Stop", "Record" {
            # "Place Window too"
            n278 = invoke class="VI" method="FP.Close"(reference=w425) -> (reference out=w424:refnum<vi>)  [unwired: 2 in, 2 out]
            n279 = invoke class="VI" method="Abort VI"(reference=w424) -> ()  [unwired: 2 in, 3 out]
          }
          frame "Playback" {
            n280 = call "Open Playback Panel.vi"("Offset"=w429, "DB VI Ref"=w430, "Playback in"=w434) -> ("Playback out"=w431:refnum<vi>)  [unwired: 8 in]
            n281 = register-events(w431, w426) -> (reference out=w433:refnum<event-registration>, error out=w432:errorcluster)  [unwired: 2 in]
          }
        }
        n282 = property on="Camera Image Right" class="ImageControl"("Image Information Shown"=w413, "Image Information Visible"=w414) -> ()  [unwired: 2 in, 2 out]
        n283 = property on="Camera Image" class="ImageControl"("Image Information Shown"=w413, "Image Information Visible"=w414) -> ()  [unwired: 2 in, 2 out]
        n284 = call <vilib>:"WPI_DashboardNT Log FieldName Cache.vi"("Operation"=enum16{"Lookup/Add", "Index", "Clear"}."Clear") -> ()  [unwired: 8 in, 3 out]
      }
      event Panel Close {
        w436 = enum32{"Stop", "Record", "Playback"}."Stop" ("Rec Mode")
        # "Playback window has been closed, abort"
        n285 = event-data() -> ()  [unwired: 1 in, 4 out]
        n286 = local write "Rec Mode"(w436) -> ()
        n287 = global write "WPI_DashboardLogging Global.vi" "Recording"(w436) -> ()
      }
      event Panel Close {
        # "Abort playback window and ourself"
        n288 = event-data() -> ()  [unwired: 1 in, 4 out]
        n289 = invoke class="VI" method="FP.Close"(reference=w440) -> (reference out=w439:refnum<vi>)  [unwired: 2 in, 2 out]
        n290 = invoke class="VI" method="Abort VI"(reference=w439) -> (error out=w438:errorcluster)  [unwired: 2 in, 2 out]
        n291 = invoke class="VI" method="Abort VI"(error in=w438) -> ()  [unwired: 2 in, 3 out]
      }
      event User Event {
        n292 = event-data() -> ("IDs"=w447:cluster{"RPC field ID":u16, "Unique ID":u16}, "String"=w446:string)  [unwired: 1 in]
        n293 = Bundle("IDs"=w447, "String"=w446) -> (w445:T8)  [unwired: 1 in]
        n294 = call <vilib>:"Retrieve RPC Response.vi"("RPC Response"=w445) -> ("Output"=w443:string[][])  [unwired: 10 in]
        n295 = Build Array (concatenate)(w441, w443) -> (w442:string[][])
        n296 = local write "Command Params"(w442) -> ()
        n297 = local write "Cmd Status"("" ("Cmd Status")) -> ()
      }
      event "Tree": Double Click {
        n298 = event-data() -> ("PlatMods"=w453:T22, "Tag"=w450:string)  [unwired: 1 in]
        n299 = Unbundle(w453) -> ("Shift"=w452:bool)  [unwired: 4 out]
        n300 = String Subset(string=w450, length (rest)=1 ("length (rest)")) -> (substring=w449:string)  [unwired: 1 in]
        n301 = Not(x=w452) -> (.not. x?=w451:bool)
        n302 = case shown="\"/\"" w449 {
          tunnel: w450 -> [_ w456]
          tunnel: w451 -> [_ w455]
          frame Default {
          }
          frame "/" {
            n303 = call <vilib>:"NT Update Persistence.vi"("Persistence"=w455, "Name"=w456) -> ()  [unwired: 9 in, 1 out]
          }
        }
      }
    }
  }
  n304 = while {
    tunnel: w65 -> [w458]
    i -> [w461]
    stop <- FALSE stop-if-true
    n305 = Wait (ms)(milliseconds to wait=u32 100) -> ()  [unwired: 1 out]
    n306 = case shown="\"Playback\"" "Rec Mode" {
      tunnel: w461 -> [_ _ w476]
      tunnel: [u32 2829099 ("Base Color") u32 11141120 ("Target Color") w465] -> w457
      frame "Stop", Default {
        # "Reset the color, extra updates don't cost much"
      }
      frame "Record" {
      }
      frame "Playback" {
        # "Playback"
        n307 = Quotient & Remainder(x=w476, y=u32 50 ("milliseconds to wait")) -> (x-y*floor(x/y)=w472:u32)  [unwired: 1 out]
        n308 = Divide(x=w472, y=u32 50 ("milliseconds to wait")) -> (x/y=w469:dbl)
        n309 = Multiply(x=6.283185307179586, y=w469) -> (x*y=w474:dbl)
        n310 = Sine(x=w474) -> (sin(x)=w473:dbl)
        n311 = Absolute Value(x=w473) -> (abs(x)=w466:dbl)
        n312 = call "Interpolate RGB Color.vi"("Proportion"=w466, "Target Color"=u32 30976, "Base Color"=u32 2829099) -> ("Result Color"=w465:u32)  [unwired: 8 in]
      }
    }
    n313 = property class="Pane"(reference=w458, "PaneColor"=w457) -> ()  [unwired: 1 in, 2 out]
  }
  n314 = local write "Dashboard Tab"(T2."Drive" ("Dashboard Tab")) -> ()
  n315 = property on="On/Off" class="Bool (strict)"("Visible"=w36) -> ()  [unwired: 2 in, 2 out]
  n316 = property on="Motor" class="Clust (strict)"("Visible"=w36) -> ()  [unwired: 2 in, 2 out]
  n317 = property on="Progress" class="Clust (strict)"("Visible"=w36) -> ()  [unwired: 2 in, 2 out]
  n318 = property on="Test Ring" class="Ring (strict)"("Visible"=w36) -> ()  [unwired: 2 in, 2 out]
  n319 = property on="Rev/Fwd" class="Clust (strict)"("Visible"=w36) -> ()  [unwired: 2 in, 2 out]
  n320 = while {
    tunnel: u16 1741 ("timeout ms (25000)") -> [w478]
    stop <- FALSE stop-if-true
    n321 = TCP Create Listener(10:w478) -> (0:w477:errorcluster, 3:w479:refnum<k5>)  [unwired: 4 in, 1 out]
    n322 = case shown="No Error" w477 {
      selector: w477 -> [w481 _]
      tunnel: w479 -> [w482 _]
      frame No Error {
        n323 = while {
          tunnel: w482 -> [w485]
          tunnel: w481 -> [w484]
          stop <- FALSE stop-if-true
          n324 = TCP Wait On Listener(8:w484, 11:w485) -> (0:w486:errorcluster, 4:w487:refnum<k5>)  [unwired: 2 in, 3 out]
          n325 = local write "TCP"(w487) -> ()
          n326 = case shown="No Error" w486 {
            frame No Error {
            }
            frame Error {
              n327 = Wait (ms)(milliseconds to wait=u32 1000) -> ()  [unwired: 1 out]
            }
          }
        }
      }
      frame Error {
        n328 = Wait (ms)(milliseconds to wait=u32 1000) -> ()  [unwired: 1 out]
      }
    }
  }
  n329 = local write "Command Selection"(u16 0 ("milliseconds to wait")) -> ()
  n330 = local write "Command Params"(string[][] [] ("Command Params")) -> ()
  n331 = global write "WPI_DashboardLogging Global.vi" "Recording"(w59) -> ()
  n332 = local write "Rec Mode"(w59) -> ()
  n333 = call <vilib>:"NT Write String.vi"("String"="Select Auto", "Name"="Auto Selector") -> ()  [unwired: 9 in, 1 out]
